vi "Get Data Channel Property - Deepth Search.vi"(8 "error in":errorcluster, 9 "Parents Section Names":string[](array[string]), 11 "Item Ref in":T1 format="%.0x") -> (0 "error out":errorcluster, 2 "Item Informations array":T2[](array[typedef]), 3 "Item Ref out":T1 format="%.0x")   [LabVIEW 2023, in "Vires VTD System Explorer.lvlib"]
uses:
  Vires VTD System Explorer.lvlib
  <vilib>/NI VeriStand/Custom Device API/Custom Device Item Ref.ctl
  Item Informations.ctl
  <vilib>/NI VeriStand/Custom Device API/Custom Device Item Info.ctl
  <vilib>/NI VeriStand/Custom Device API/Custom Device Channel.ctl
  <vilib>/NI VeriStand/Custom Device API/Custom Device Channel Type.ctl
  Data Channel Custom Property.ctl
  <vilib>/NI VeriStand/Custom Device Tools/Custom Device Utility Library/Custom Device Utility Library.lvlib
  <vilib>/NI VeriStand/Custom Device API/Custom Device API.lvlib
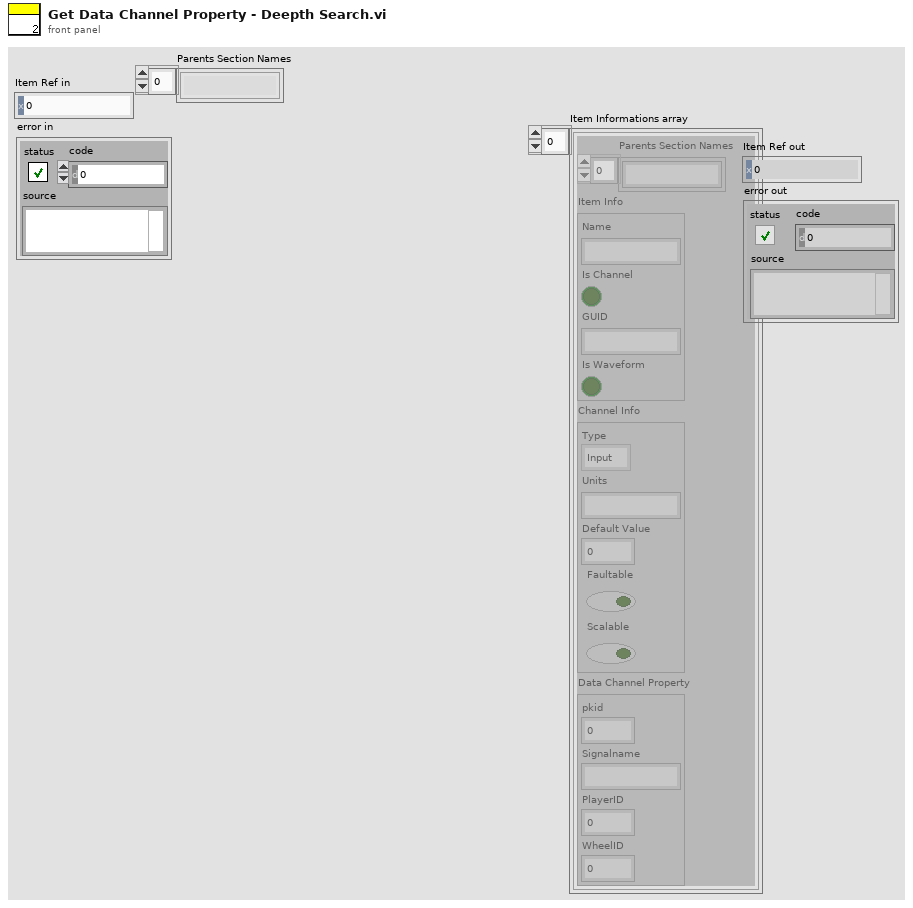
[diagram p1: front panel]
types:
  T1 = typedef "Custom Device API.lvlib/Custom Device Item Ref.ctl" = u64
  T2 = typedef "Vires VTD System Explorer.lvlib/Item Informations.ctl" = cluster{"Parents Section Names":string[], "Item Info":T3, "Channel Info":T4, "Data Channel Property":T6}
  T3 = typedef "Custom Device API.lvlib/Custom Device Item Info.ctl" = cluster{"Name":string, "Is Channel":bool, "GUID":string, "Is Waveform":bool}
  T4 = typedef "Custom Device API.lvlib/Custom Device Channel.ctl" = cluster{"Type":T5, "Units":string, "Default Value":dbl, "Faultable":bool, "Scalable":bool}
  T5 = typedef "Custom Device API.lvlib/Custom Device Channel Type.ctl" = enum16{"Input", "Output"}
  T6 = typedef "Vires VTD System Explorer.lvlib/Data Channel Custom Property.ctl" = cluster{"pkid":u32, "Signalname":string, "PlayerID":u8, "WheelID":i32}
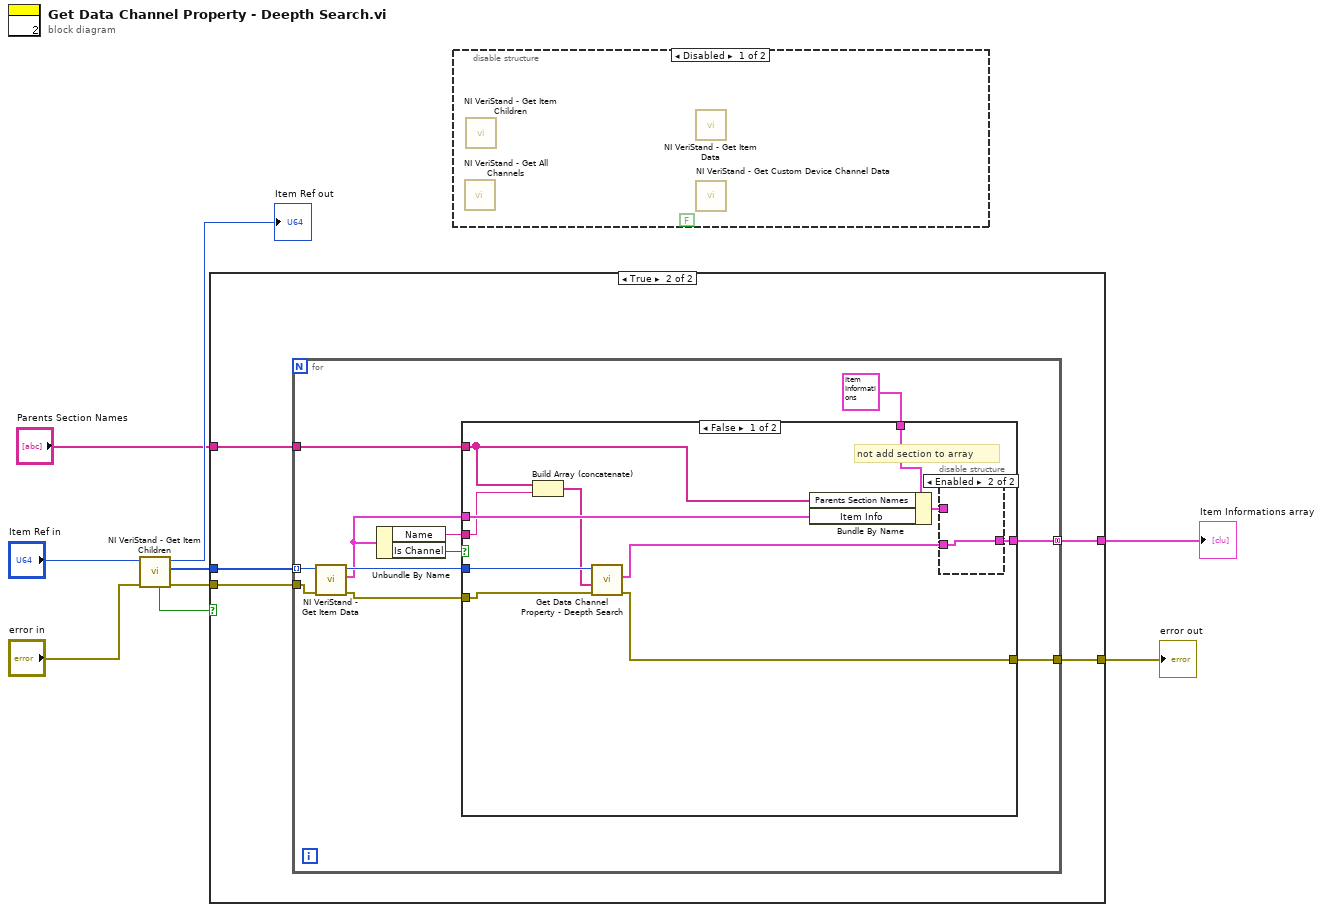
[diagram p0: block diagram]
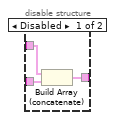
[diagram p3: hidden frame]
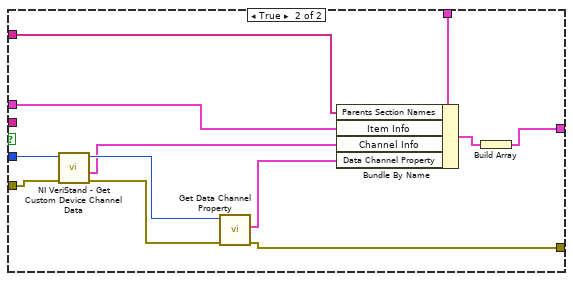
[diagram p4: hidden frame]
diagram:
  n1 = call <vilib>:"NI VeriStand - Get Item Children.vi"("error in (no error)"="error in", "Item Ref in"="Item Ref in") -> ("error out"=w4:errorcluster, "Child Refs"=w8:T1[], "Item Ref out"=→"Item Ref out":T1, "Found"=w9:bool)  [unwired: 6 in]
  n2 = case shown="True" w9 {
    tunnel: w8 -> [_ w14]
    tunnel: [_ w13] -> w2
    tunnel: w4 -> [_ w12]
    tunnel: [_ w11] -> w3
    tunnel: "Parents Section Names" -> [_ w10]
    frame False {
    }
    frame True {
      n3 = for {
        tunnel: w14 -> [w25] mode=indexing
        tunnel: [w21] -> w13 mode=concatenating
        tunnel: w12 -> [w20]
        tunnel: [w18] -> w11
        tunnel: w10 -> [w15]
        n4 = call <vilib>:"NI VeriStand - Get Item Data.vi"("error in (no error)"=w20, "Item Ref in"=w25) -> ("error out"=w19:errorcluster, "Item Info"=w22:T3, "Item Ref out"=w23:T1)  [unwired: 6 in, 1 out]
        n5 = Unbundle By Name(w22) -> ("Name"=w16:string, "Is Channel"=w24:bool)
        n6 = case shown="False" w24 {
          tunnel: w23 -> [w32 w42]
          tunnel: w22 -> [w33 w51]
          tunnel: [w26 w47] -> w21
          tunnel: w19 -> [w36 w44]
          tunnel: [w35 w43] -> w18
          tunnel: T2 {"Parents Section Names"=[], "Item Info"={"Name"="", "Is Channel"=FALSE, "GUID"="", "Is Waveform"=FALSE}, "Channel Info"={"Type"=enum."Input", "Units"="", "Default Value"=0.0, "Faultable"=FALSE, "Scalable"=FALSE}, "Data Channel Property"={"pkid"=0, "Signalname"="", "PlayerID"=1, "WheelID"=0}} ("Item Informations") -> [w34 w45]
          tunnel: w16 -> [w31 _]
          tunnel: w15 -> [w28 w41]
          frame False {
            # "not add section to array"
            n7 = Build Array (concatenate)(w28, w31) -> (w30:string[])
            n8 = call "Get Data Channel Property - Deepth Search.vi"("error in"=w36, "Parents Section Names"=w30, "Item Ref in"=w32) -> ("error out"=w35:errorcluster, "Item Informations array"=w27:T2[])  [unwired: 6 in, 1 out]
            n9 = Bundle By Name(cluster=w34, "Parents Section Names"=w28, "Item Info"=w33) -> (w29:T2)
            n10 = disable-structure shown="Enabled" {
              disable-tunnel: w29 -> [w39 _]
              disable-tunnel: w27 -> [w38 w40]
              disable-tunnel: [w37 w40] -> w26
              frame Disabled {
                n11 = Build Array (concatenate)(w39, w38) -> (w37:T2[])
              }
              frame Enabled {
              }
            }
          }
          frame True {
            n12 = call <vilib>:"NI VeriStand - Get Custom Device Channel Data.vi"("error in (no error)"=w44, "Channel Ref in"=w42) -> ("error out"=w46:errorcluster, "Channel"=w50:T4, "Channel Ref out"=w52:T1)  [unwired: 4 in, 3 out]
            n13 = call "Get Data Channel Property.vi"("error in (no error)"=w46, "Item Ref in"=w52) -> ("error out"=w43:errorcluster, "Data Channel Property"=w49:T6)  [unwired: 7 in, 1 out]
            n14 = Bundle By Name(cluster=w45, "Parents Section Names"=w41, "Item Info"=w51, "Channel Info"=w50, "Data Channel Property"=w49) -> (w48:T2)
            n15 = Build Array(w48) -> (w47:T2[])
          }
        }
      }
    }
  }
  "Item Informations array" <- w2
  "error out" <- w3
  n16 = disable-structure shown="Disabled" {
    frame Disabled {
      (unwired) FALSE ("Found")
      n17 = call <vilib>:"NI VeriStand - Get All Channels.vi"() -> ()  [unwired: 8 in, 4 out]
      n18 = call <vilib>:"NI VeriStand - Get Item Children.vi"() -> ()  [unwired: 8 in, 4 out]
      n19 = call <vilib>:"NI VeriStand - Get Item Data.vi"() -> ()  [unwired: 8 in, 4 out]
      n20 = call <vilib>:"NI VeriStand - Get Custom Device Channel Data.vi"() -> ()  [unwired: 6 in, 6 out]
    }
    frame Enabled {
    }
  }
